vi "FGV_Timer.vi"(7 "action":enum16{"reset", "get"}(ring)=enum."get", 10 "target":dbl) -> (2 "time":dbl, 3 "time has elapsed?":bool)   [LabVIEW 2019]
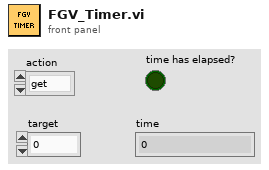
[diagram p1: front panel]
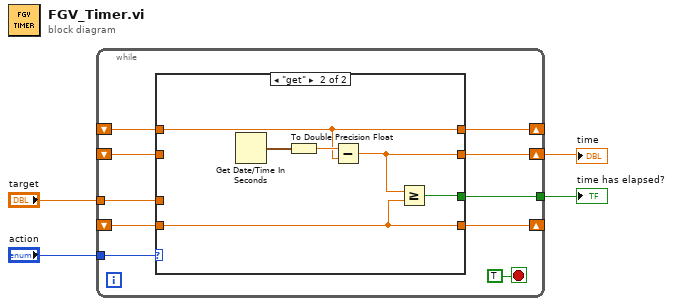
[diagram p0: block diagram]
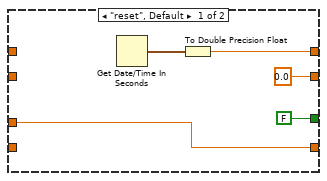
[diagram p2: hidden frame]
diagram:
  n1 = while {
    tunnel: "action" -> [w14]
    tunnel: "target" -> [w13]
    shift-right: [w11] -> _
    shift-left: _ -> [w10]
    shift-right: [w9] -> w2
    shift-left: _ -> [w8]
    tunnel: [w7] -> w1
    shift-right: [w6] -> _
    shift-left: _ -> [w5]
    stop <- TRUE stop-if-true
    n2 = case shown="\"get\"" w14 {
      tunnel: w13 -> [w15 _]
      tunnel: [w18 w23] -> w11
      tunnel: w10 -> [_ w23]
      tunnel: [0.0 ("double precision float") w22] -> w9
      tunnel: w8 -> [_ _]
      tunnel: [FALSE w21] -> w7
      tunnel: [w15 w20] -> w6
      tunnel: w5 -> [_ w20]
      frame "reset", Default {
        n3 = Get Date/Time In Seconds() -> (seconds since 1Jan1904=w19:timestamp)
        n4 = To Double Precision Float(number=w19) -> (double precision float=w18:dbl)
      }
      frame "get" {
        n5 = Get Date/Time In Seconds() -> (seconds since 1Jan1904=w24:timestamp)
        n6 = To Double Precision Float(number=w24) -> (double precision float=w25:dbl)
        n7 = Subtract(x=w25, y=w23) -> (x-y=w22:dbl)
        n8 = Greater Or Equal?(x=w22, y=w20) -> (x >= y?=w21:bool)
      }
    }
  }
  "time" <- w2
  "time has elapsed?" <- w1
